vi "Set Notifier Ref.vi"(8 "error in (no error)":errorcluster, 10 "notifier in":refnum<notifier>, 11 "CVT_String in":refnum<class "CVT_String.lvclass">) -> (0 "error out":errorcluster, 3 "CVT_String out":refnum<class "CVT_String.lvclass">)   [LabVIEW 2024, in "Current Value Table.lvlib" / "CVT_String.lvclass"]
uses:
  CVT_String.lvclass
  CVT_String.lvclass/CVT_String.ctl
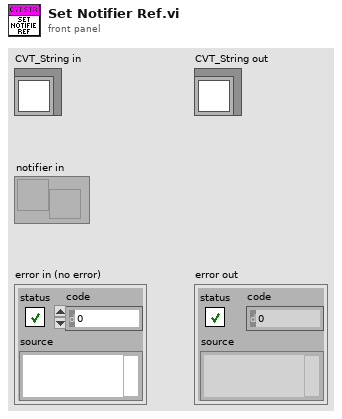
[diagram p1: front panel]
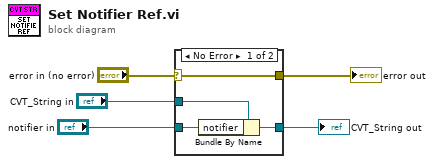
[diagram p0: block diagram]
diagram:
  n1 = case shown="No Error" "error in (no error)" {
    selector: "error in (no error)" -> [w9 w11]
    tunnel: [w9 w11] -> w4
    tunnel: [w7 w10] -> w2
    tunnel: "CVT_String in" -> [w8 w10]
    tunnel: "notifier in" -> [w6 _]
    frame No Error {
      n2 = Bundle By Name(cluster=w8, "notifier"=w6) -> (w7:refnum<class "CVT_String.lvclass">)
    }
    frame Error {
    }
  }
  "error out" <- w4
  "CVT_String out" <- w2
